vi "20150818 UL sensor+servo test.vi"() -> ()   [LabVIEW 2013]
uses:
  <vilib>/MakerHub/LINX/Public/Sensors/Motion/Servo/Servo Open N Channels.vi
  <vilib>/MakerHub/LINX/Public/Sensors/Motion/Servo/Servo Close N Channels.vi
  <vilib>/MakerHub/LINX/Public/Sensors/Motion/Servo/Servo Set Pulse Width N Channels.vi
  <vilib>/MakerHub/LINX/LMH-LINX.lvlib
  <vilib>/MakerHub/LINX/Public/Sensors/Motion/Servo/Servo.lvlib
  <vilib>/MakerHub/LINX/Public/Sensors/Ultrasonic/Ultrasonic.lvlib
panel:
  out "Centimeters":dbl=13.424440505523
  in  "Servo Channels":u8[](array[numeric])=[2, 3, 4, 5, 6, 7, 8, 9, 10, 11, 12, 13]
  in  "error in (no error)":errorcluster
  out "Error Out":errorcluster
  out "Initialize OK?":bool=TRUE
  in  "Stop Button":bool
  in  "Pulse Widths (uS)":u16[](array[numeric])=[1500, 1100, 1100, 1500, 1800, 1700, 1500, 1700, 1500, 1500, 1000, 1200] min=600 max=2400 step=100
  in  "Serial Port":refnum<visa-resource-name>="COM10"
  # "up: CK"
  # "up: CK"
  # "up: CCK"
  # "up: CK"
  # "up: CK"
  # "up: CCK"
  # "up: CK"
  # "up: CK"
  # "up: CCK"
  # "up: CK"
  # "up: CK"
  # "up: CCK"
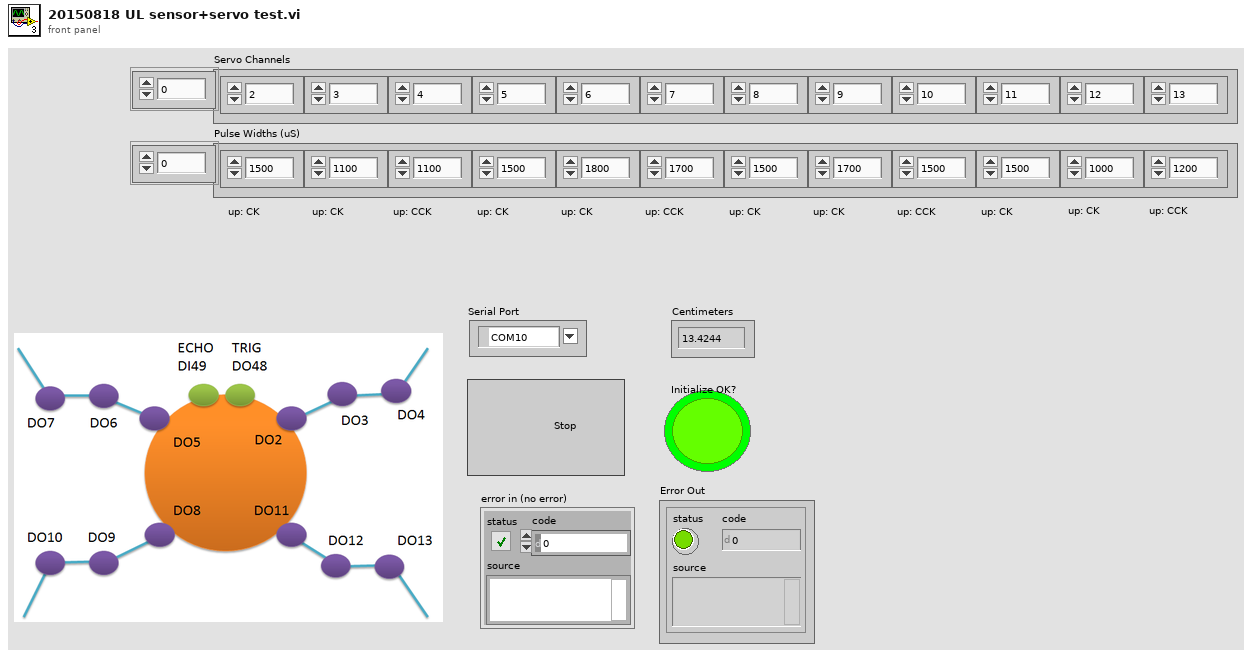
[diagram p1: front panel]
types:
  T1 = typedef "LMH-LINX.lvlib/LINX Ref.ctl" = cluster{"Platform":T2, "Interface":T3, "LINX Device Config":T4}
  T2 = typedef "LMH-LINX.lvlib/Platform.ctl" = enum16{"LINX", "myRIO"}
  T3 = typedef "LMH-LINX.lvlib/Interface.ctl" = enum16{"Serial", "TCP"}
  T4 = typedef "LMH-LINX.lvlib/Device.lvlib/LINX Device Config.ctl" = cluster{"Interface":T3, "COM Port":refnum<visa-resource-name>, "TCP Configuration":T5, "Device Family":u8, "Device ID":u8, "Device Name":string, "TCP Ref":refnum<k5>, "Channels":T6}
  T5 = typedef "LMH-LINX.lvlib/Device.lvlib/TCP Config.ctl" = cluster{"IP Address":string, "Port":u16}
  T6 = typedef "LMH-LINX.lvlib/Channels.ctl" = cluster{"DI":u8[], "DO":u8[], "AI":u8[], "AO":u8[], "PWM":u8[], "QE":u8[], "UART":u8[], "I2C 2":u8[], "SPI":u8[], "CAN":u8[], "Servo":u8[], "AI Ref (V)":dbl, "AO Ref (V)":dbl, "AO Resolution (Bits)":u8}
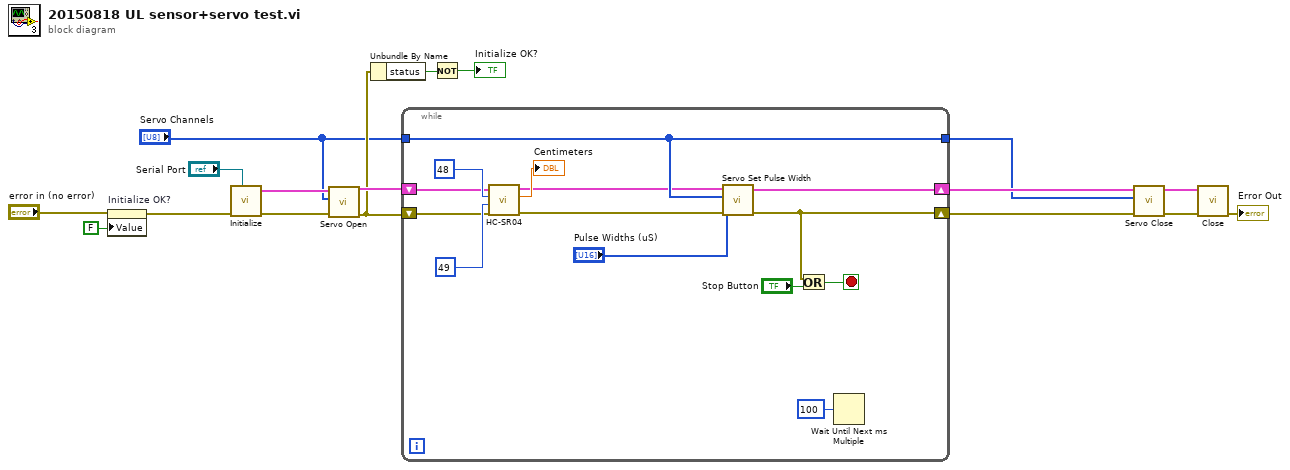
[diagram p0: block diagram]
diagram:
  n1 = property on="Initialize OK?" class="Bool (strict)"(error in="error in (no error)", "Value"=FALSE ("Initialize OK?")) -> (error out=w6:errorcluster)  [unwired: 1 in, 1 out]
  n2 = call <vilib>:"Initialize.vi"("Serial Port"="Serial Port", "Error In"=w6) -> ("Error Out"=w16:errorcluster, "LINX Ref"=w15:T1)  [unwired: 7 in, 1 out]
  n3 = call-poly <vilib>:"Servo Open.vi"("Error In"=w16, "Servo Channels"="Servo Channels", "LINX Resource"=w15) -> ("Error Out"=w9:errorcluster, "LINX Resource"=w14:T1)  [unwired: 7 in]
  n4 = Unbundle By Name(w9) -> ("status"=w8:bool)
  n5 = while {
    shift-right: [w29] -> w10
    shift-left: w9 -> [w20]
    tunnel: "Servo Channels" -> [w27]
    shift-right: [w28] -> w13
    shift-left: w14 -> [w22]
    tunnel: [w27] -> w1
    stop <- w31 stop-if-true
    n6 = call <vilib>:"HC-SR04.vi"("Error In"=w20, "Echo Pin (DI)"=u8 49, "Trig"=u8 48, "LINX Resource"=w22) -> ("Error Out"=w19:errorcluster, "Centimeters"=→"Centimeters":dbl, "LINX Resource"=w21:T1)  [unwired: 4 in, 1 out]
    n7 = call-poly <vilib>:"Servo Set Pulse Width.vi"("Error In"=w19, "Pulse Widths (uS)"="Pulse Widths (uS)", "Servo Channels"=w27, "LINX Resource"=w21) -> ("Error Out"=w29:errorcluster, "LINX Resource"=w28:T1)  [unwired: 6 in]
    n8 = Or(x=w29, y="Stop Button") -> (x .or. y?=w31:bool)
    n9 = Wait Until Next ms Multiple(millisecond multiple=u32 100) -> ()  [unwired: 1 out]
  }
  n10 = Not(x=w8) -> (.not. x?=→"Initialize OK?":bool)
  n11 = call-poly <vilib>:"Servo Close.vi"("Error In"=w10, "Servo Channels"=w1, "LINX Resource"=w13) -> ("Error Out"=w11:errorcluster, "LINX Resource"=w12:T1)  [unwired: 7 in]
  n12 = call <vilib>:"Close.vi"("Error In"=w11, "LINX Resource"=w12) -> ("Error Out"=→"Error Out":errorcluster)  [unwired: 8 in, 1 out]
